vi "LSCI332 Zone Setup.vi"(4 "Zones":T1(array[cluster])=[{"TempFin"=400.0, "P"=1000.0, "I"=0.0, "D"=0, "ManualOutput(%)"=0.0, "Range"=5}, {"TempFin"=400.0, "P"=1000.0, "I"=0.0, "D"=0, "ManualOutput(%)"=0.0, "Range"=5}, {"TempFin"=400.0, "P"=1000.0, "I"=0.0, "D"=0, "ManualOutput(%)"=0.0, "Range"=5}, {"TempFin"=400.0, "P"=1000.0, "I"=0.0, "D"=0, "ManualOutput(%)"=0.0, "Range"=5}, {"TempFin"=400.0, "P"=1000.0, "I"=0.0, "D"=0, "ManualOutput(%)"=0.0, "Range"=5}, {"TempFin"=400.0, "P"=1000.0, "I"=0.0, "D"=0, "ManualOutput(%)"=0.0, "Range"=5}, {"TempFin"=400.0, "P"=1000.0, "I"=0.0, "D"=0, "ManualOutput(%)"=0.0, "Range"=5}, {"TempFin"=400.0, "P"=1000.0, "I"=0.0, "D"=0, "ManualOutput(%)"=0.0, "Range"=5}, {"TempFin"=400.0, "P"=1000.0, "I"=0.0, "D"=0, "ManualOutput(%)"=0.0, "Range"=5}, {"TempFin"=400.0, "P"=1000.0, "I"=0.0, "D"=0, "ManualOutput(%)"=0.0, "Range"=5}] {"D" max=1000 step=1; "I" min=0.0 max=1000.0 step=0.1 format="%#.1f"; "Range" max=5 step=1; "ManualOutput(%)" min=-100.0 max=100.0 step=0.01 format="%#.2g"; "P" min=0.0 max=1000.0 step=0.1 format="%#.1f"; "TempFin" min=0.0 max=400.0 step=0.001 format="%#.3g"}, 11 "error in":errorcluster) -> (15 "error out":errorcluster)   [LabVIEW 2019]
doc: "Ce Vi permet la configuration des zones de contrôles ainsi que la gestion de leures différents paramètres. À l'ouverture, le VI lit et retourne les paramètres de zones actuels"
uses:
  <vilib>/Utility/error.llb/DialogType.ctl
panel:
  in  "Écrire":bool
  in  "VISA Rsrc":refnum<visa-resource-name>="GPIB0::12::INSTR" caption="Adresse du contrôlleur"
  in  "Quit":bool
  # "Zones"
  # "Paramètres"
  # "1"
  # "2"
  # "3"
  # "4"
  # "5"
  # "6"
  # "7"
  # "8"
  # "9"
  # "10"
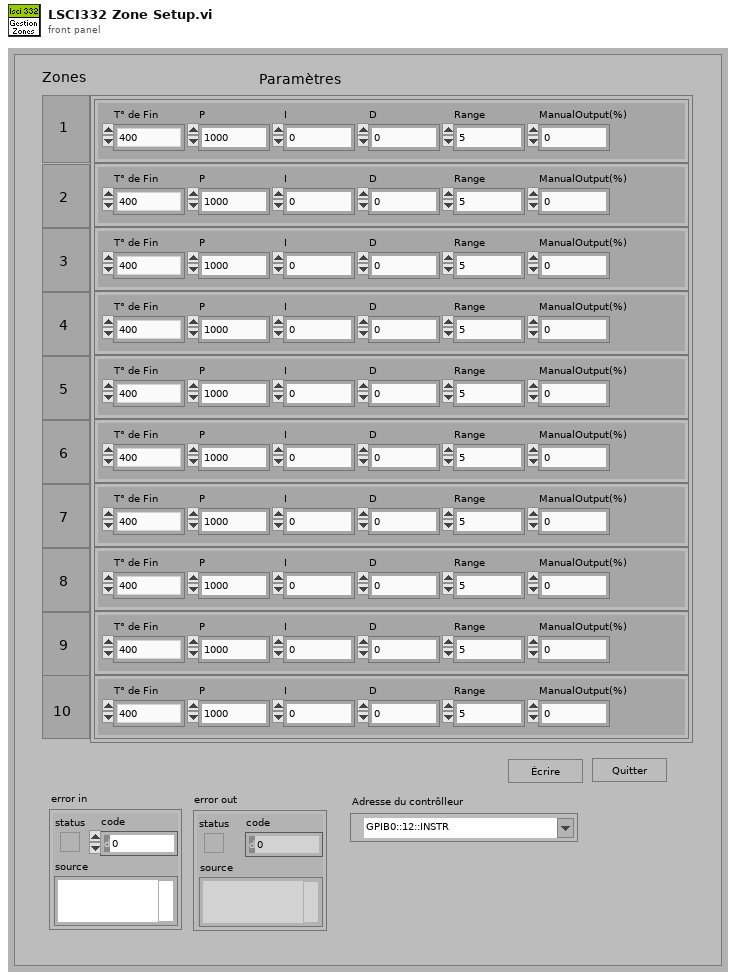
[diagram p1: front panel]
types:
  T1 = cluster{"TempFin":dbl, "P":dbl, "I":dbl, "D":u32, "ManualOutput(%)":dbl, "Range":u32}[]
  T2 = cluster{"TempFin":dbl, "P":dbl, "I":dbl, "D":u32, "ManualOutput(%)":dbl, "Range":u32}
  T3 = typedef "DialogType.ctl" = u16
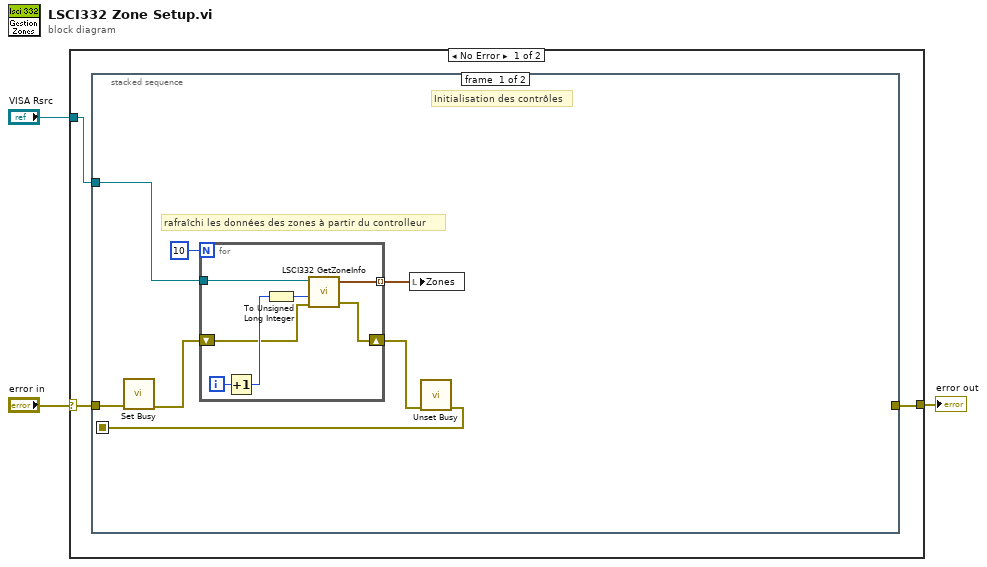
[diagram p0: block diagram]
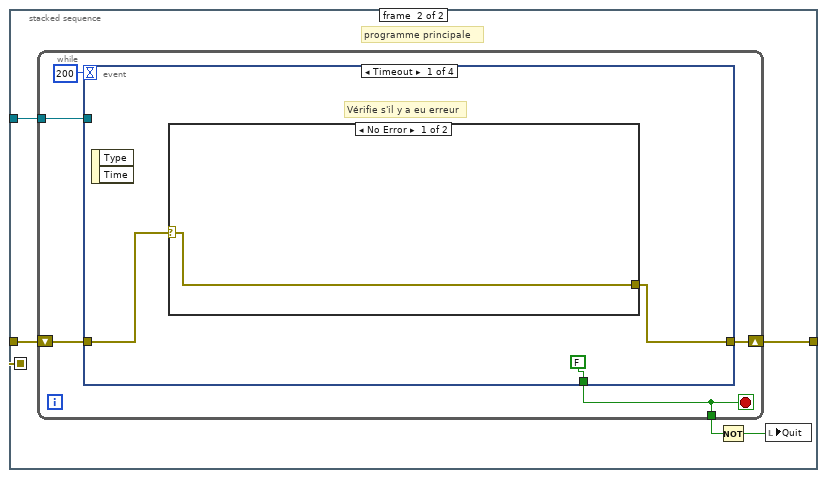
[diagram p2: hidden frame]
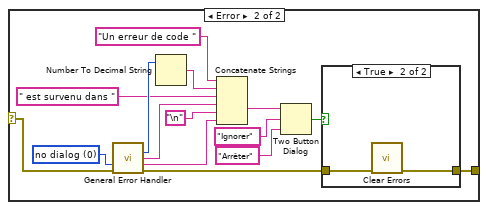
[diagram p3: hidden frame]
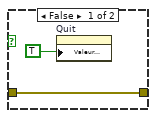
[diagram p4: hidden frame]
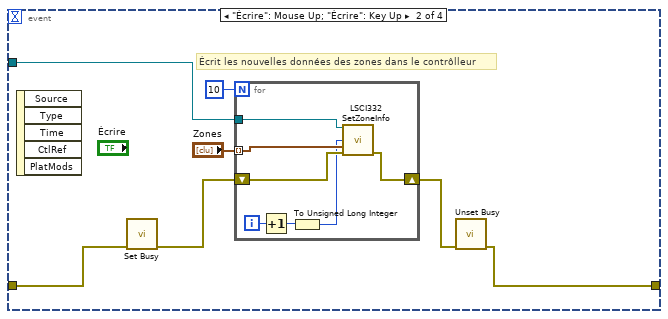
[diagram p5: hidden frame]
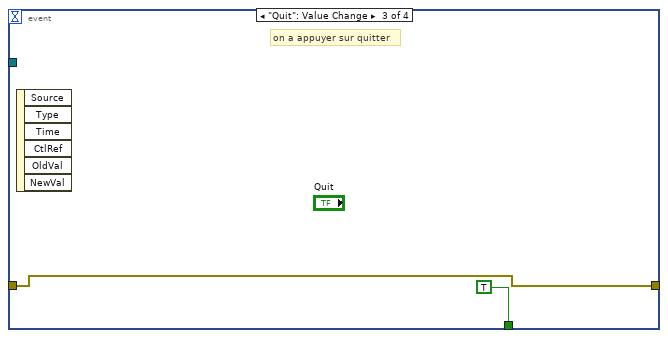
[diagram p6: hidden frame]
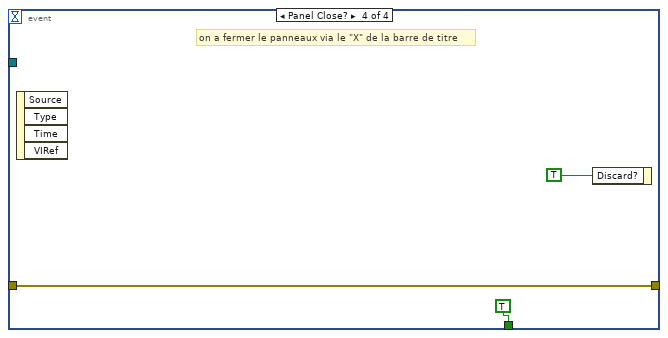
[diagram p7: hidden frame]
diagram:
  n1 = case shown="No Error" "error in" {
    selector: "error in" -> [w6 w73]
    tunnel: [w4 w73] -> w2
    tunnel: "VISA Rsrc" -> [w5 _]
    frame No Error {
      n2 = stacked-sequence {
        seq-local: [w12 _] -> [_ w21]
        tunnel: w6 -> [w13 _]
        tunnel: w5 -> [w10 w25]
        tunnel: [_ w24] -> w4
        frame #0 {
          # "rafraîchi les données des zones à partir du controlleur"
          # "Initialisation des contrôles"
          n3 = call <vilib>:"Set Busy.vi"("error in (no error)"=w13) -> ("error out"=w9:errorcluster)  [unwired: 9 in, 1 out]
          n4 = for {
            N: 10 -> [_]
            tunnel: w10 -> [w17]
            shift-right: [w15] -> w8
            shift-left: w9 -> [w16]
            tunnel: [w14] -> w7 mode=indexing
            i -> [w20]
            n5 = Increment(x=w20) -> (x+1=w19:i32)
            n6 = To Unsigned Long Integer(number=w19) -> (unsigned 32bit integer=w18:u32)
            n7 = call <userlib>:"LSCI332 GetZoneInfo.vi"("error in (no error)"=w16, "Zone"=w18, "VISA Rsrc"=w17) -> ("error out"=w15:errorcluster, "Paramètres"=w14:T2)  [unwired: 6 in]
          }
          n8 = local write "Zones"(w7) -> ()
          n9 = call <vilib>:"Unset Busy.vi"("error in (no error)"=w8) -> ("error out"=w12:errorcluster)  [unwired: 10 in]
        }
        frame #1 {
          # "programme principale"
          n10 = while {
            shift-right: [w28] -> w24
            shift-left: w21 -> [w29]
            tunnel: w25 -> [w27]
            tunnel: [w26] -> w23
            stop <- w26 stop-if-true
            n11 = event shown="[0] Timeout" {
              selector: _ -> [_ _ _ _]
              dyn-events: _ -> [_ _ _ _]
              timeout: 200 -> [_ _ _ _]
              tunnel: w29 -> [w33 w57 w68 w70]
              tunnel: [w32 w54 w68 w70] -> w28
              tunnel: w27 -> [_ w58 _ _]
              tunnel: [FALSE _ TRUE TRUE] -> w26
              event Timeout {
                # "Vérifie s'il y a eu erreur"
                n12 = event-data() -> ()  [unwired: 1 in, 2 out]
                n13 = case shown="No Error" w33 {
                  selector: w33 -> [w34 w35]
                  tunnel: [w34 w36] -> w32
                  frame No Error {
                  }
                  frame Error {
                    w46 = T3 0 items=["no dialog", "OK message", "continue or stop message", "OK message + warnings", "continue/stop + warnings"] ("type of dialog (OK msg:1)")
                    n14 = call <vilib>:"General Error Handler.vi"("type of dialog (OK msg:1)"=w46, "error in (no error)"=w35) -> ("code out"=w42:i32, "source out"=w41:string, "message"=w39:string, "error out"=w37:errorcluster)  [unwired: 9 in, 1 out]
                    n15 = Number To Decimal String(number=w42) -> (decimal integer string=w43:string)  [unwired: 1 in]
                    n16 = Concatenate Strings("Un erreur de code " ("string"), w43, " est survenu dans " ("string"), w41, "\n", w39) -> (w38:string)
                    n17 = Two Button Dialog(message=w38, 1:"Arrêter" ("F button name (\"Cancel\")"), 2:"Ignorer" ("T button name (\"OK\")")) -> (T button?=w49:bool)
                    n18 = case shown="True" w49 {
                      tunnel: w37 -> [w51 w52]
                      tunnel: [w51 w53] -> w36
                      frame False {
                        n19 = property on="Quit" class="Bool (strict)"("Valeur (Signalisation)"=TRUE ("Value (Signaling)")) -> ()  [unwired: 2 in, 2 out]
                      }
                      frame True {
                        n20 = call <vilib>:"Clear Errors.vi"("error in (no error)"=w52) -> ("error out"=w53:errorcluster)  [unwired: 5 in, 1 out]
                      }
                    }
                  }
                }
              }
              event "Écrire": Mouse Up; "Écrire": Key Up {
                # "Écrit les nouvelles données des zones dans le contrôlleur"
                n21 = event-data() -> ()  [unwired: 1 in, 5 out]
                n22 = call <vilib>:"Set Busy.vi"("error in (no error)"=w57) -> ("error out"=w56:errorcluster)  [unwired: 9 in, 1 out]
                n23 = for {
                  N: 10 -> [_]
                  tunnel: w58 -> [w62]
                  shift-right: [w61] -> w59
                  shift-left: w56 -> [w66]
                  tunnel: "Zones" -> [w65] mode=indexing
                  i -> [w67]
                  n24 = Increment(x=w67) -> (x+1=w64:i32)
                  n25 = To Unsigned Long Integer(number=w64) -> (unsigned 32bit integer=w63:u32)
                  n26 = call <userlib>:"LSCI332 SetZoneInfo.vi"("VISA Rsrc"=w62, "Zone"=w63, "Paramètres"=w65, "error in (no error)"=w66) -> ("error out"=w61:errorcluster)  [unwired: 11 in]
                }
                n27 = call <vilib>:"Unset Busy.vi"("error in (no error)"=w59) -> ("error out"=w54:errorcluster)  [unwired: 10 in]
              }
              event "Quit": Value Change {
                # "on a appuyer sur quitter"
                n28 = event-data() -> ()  [unwired: 1 in, 6 out]
              }
              event Panel Close? {
                # "on a fermer le panneaux via le \"X\" de la barre de titre"
                n29 = event-data() -> ()  [unwired: 1 in, 4 out]
                n30 = event-data("Discard?"=TRUE) -> ()  [unwired: 1 in, 1 out]
              }
            }
          }
          n31 = Not(x=w23) -> (.not. x?=w22:bool)
          n32 = local write "Quit"(w22) -> ()
        }
      }
    }
    frame Error {
    }
  }
  "error out" <- w2
